vi "Main.vi"() -> ()   [LabVIEW 2013]
uses:
  <vilib>/myRIO/Instrument Drivers/Onboard IO/I2C/typedefs/I2C User Configuration.ctl
  <vilib>/myRIO/Instrument Drivers/Onboard IO/I2C/typedefs/I2C Transfer Rate.ctl
  <vilib>/Platform/TimedLoop/XDataNode/timing_clust.ctl
  <vilib>/Platform/TimedLoop/XDataNode/nitl_modes.ctl
  <vilib>/Platform/TimedLoop/XDataNode/wakeup.ctl
  <vilib>/myRIO/Common/Instrument Driver Framework/myRIO v1.0/DIO/vis/myRIO v1.1 Open DIO.vi
  <vilib>/myRIO/Common/Instrument Driver Framework/myRIO v1.0/I2C/vis/myRIO v1.1 Open I2C.vi
  <vilib>/myRIO/Common/Instrument Driver Framework/myRIO v1.0/UART/vis/myRIO v1.0 Close UART.vi
  <vilib>/myRIO/Common/Instrument Driver Framework/Utilities/vis/Validate Channels.vi
  <vilib>/myRIO/Common/Instrument Driver Framework/myRIO v1.0/DIO/vis/myRIO v1.0 Reserve DIO.vi
  <vilib>/myRIO/Common/Instrument Driver Framework/myRIO v1.0/I2C/vis/myRIO v1.0 Reserve I2C.vi
  <vilib>/myRIO/Common/Instrument Driver Framework/myRIO v1.0/Resource Manager/vis/myRIO v1.0 Reserve Channel List.vi
  <vilib>/myRIO/Common/Instrument Driver Framework/myRIO v1.0/DIO/vis/myRIO v1.0 Build MUX Configuration DIO.vi
  <vilib>/myRIO/Common/Instrument Driver Framework/myRIO v1.0/I2C/vis/myRIO v1.0 Build MUX Configuration I2C.vi
  <vilib>/myRIO/Common/Instrument Driver Framework/myRIO v1.0/Resource Manager/vis/myRIO v1.0 Reserve Channel.vi
  <vilib>/myRIO/Common/Instrument Driver Framework/myRIO v1.0/Resource Manager/vis/myRIO v1.0 Unreserve Channel.vi
  <vilib>/myRIO/Common/Instrument Driver Framework/myRIO v1.0/Resource Manager/vis/myRIO v1.0 Create Configuration List.vi
  <vilib>/myRIO/Common/Instrument Driver Framework/myRIO v1.0/Resource Manager/vis/myRIO v1.0 Build Mutex Name.vi
  <vilib>/myRIO/Common/Instrument Driver Framework/myRIO v1.0/myRIO v1.1 Open.vi
  <vilib>/Utility/VariantDataType/GetNumericInfo.vi
  <vilib>/Utility/error.llb/Error Cluster From Error Code.vi
  <vilib>/myRIO/Common/Instrument Driver Framework/Utilities/vis/IO Manager.vi
  <vilib>/myRIO/Common/Instrument Driver Framework/Utilities/vis/Configuration Manager.vi
  <vilib>/myRIO/Common/Instrument Driver Framework/myRIO v1.0/Resource Manager/vis/myRIO v1.0 Configure IO.vi
  <vilib>/myRIO/Common/Instrument Driver Framework/myRIO v1.0/myRIO v1.0 Close.vi
  <vilib>/myRIO/Common/Instrument Driver Framework/myRIO v1.0/I2C/vis/myRIO v1.0 Configure I2C.vi
  <vilib>/myRIO/Common/Instrument Driver Framework/myRIO v1.0/I2C/vis/myRIO v1.0 Write I2C.vi
  <vilib>/myRIO/Common/Instrument Driver Framework/myRIO v1.0/DIO/vis/myRIO v1.0 Read DIO.vi
  <vilib>/myRIO/Common/Instrument Driver Framework/myRIO v1.0/DIO/vis/myRIO v1.0 Write DIO.vi
  <vilib>/myRIO/Common/Instrument Driver Framework/myRIO v1.0/I2C/vis/myRIO v1.0 Read I2C.vi
  <vilib>/myRIO/Common/Instrument Driver Framework/Utilities/vis/FPGA Ref Manager.vi
  <vilib>/myRIO/Common/Instrument Driver Framework/myRIO v1.0/myRIO v1.0 Reset FPGA.vi
  <vilib>/platform/TimedLoop/XDataNode/XDataNode.xnode
  <vilib>/myRIO/Instrument Drivers/Utilities/Utilities.lvlib
  <vilib>/myRIO/Instrument Drivers/Onboard IO/I2C/I2C.lvlib
  <vilib>/myRIO/Instrument Drivers/Onboard IO/DIO/DIO.lvlib
  <vilib>/Platform/TimedLoop/XDataNode/XDNodeRunTimeDep.lvlib
panel:
  out "INT_SOURCE":bool[](array[boolean])
  out "Waveform Chart":cluster{i16, i16, i16}(graph)
  out "DATA":u8[](array[numeric]) format="%02x"
  out "Z":i16
  out "Y":i16
  out "X":i16
  in  "[ESC]":bool
  # "Accelerometer demo"
  # "DATAX0"
  # "DATAX1"
  # "DATAY0"
  # "DATAY1"
  # "DATAZ0"
  # "DATAZ1"
  # "D = data ready\n1T = single-tap\n2T = double-tap"
  # "A = activity\nI = inactivity\nF = free fall"
  # "W = watermark\nO = overrun"
  # "D   1T  2T   A    I     F    W   O"
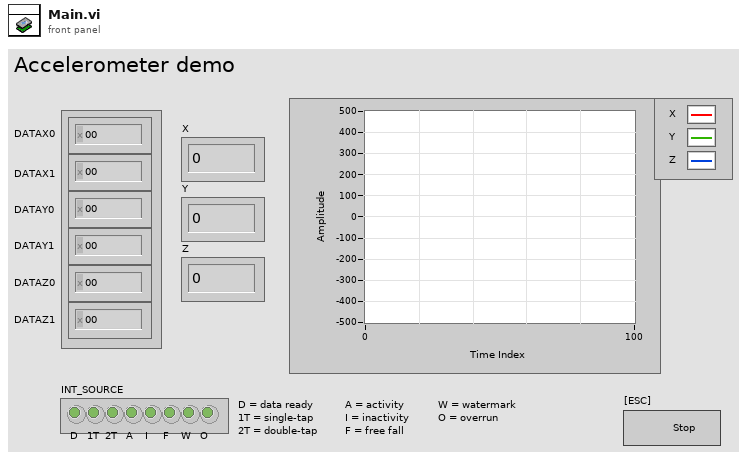
[diagram p1: front panel]
types:
  T1 = typedef "I2C.lvlib/I2C User Configuration.ctl" = cluster{"I2C Transfer Rate":T2}
  T2 = typedef "I2C.lvlib/I2C Transfer Rate.ctl" = enum16{"Standard Mode (100 kbps)", "Fast Mode (400 kbps)"}
  T3 = typedef "I2C.lvlib/I2C Reference.ctl" = cluster{"myRIO Reference":T4, "I2C Channels Enum":T8, "I2C Configuration":T9}
  T4 = typedef "myRIO Generic Hardware Reference.ctl" = cluster{"myRIO Model":T5, "myRIO Hardware Reference":T6}
  T5 = typedef "Hardware Version Enum.ctl" = enum16{"Unknown", "myRIO-1900", "myRIO-1950"}
  T6 = typedef "myRIO v1.0 Reference.ctl" = cluster{"Generic FPGA Reference":T7, "Allow multiple opens":bool}
  T7 = typedef "Generic FPGA Reference.ctl" = refnum<k20>
  T8 = typedef "I2C Channels Enum.ctl" = enum16{"Not Connected", "A/I2C", "B/I2C"}
  T9 = typedef "I2C.lvlib/I2C Configuration.ctl" = cluster{"I2C Transfer Rate":T2}
  T10 = typedef "DIO.lvlib/DIO Reference.ctl" = cluster{"myRIO Reference":T4, "DIO Channels List":T11}
  T11 = typedef "DIO Channels List.ctl" = T12[]
  T12 = typedef "DIO Channels Enum.ctl" = enum16{"Not Connected", "C/DIO0", "C/DIO1", "C/DIO2", "C/DIO3", "C/DIO4", "C/DIO5", "C/DIO6", "C/DIO7", "A/DIO0", "A/DIO1", "A/DIO2", "A/DIO3", "A/DIO4", "A/DIO5", "A/DIO6", "A/DIO7", "A/DIO8", "A/DIO9", "A/DIO10", "A/DIO11", "A/DIO12", "A/DIO13", "A/DIO14", "A/DIO15", "B/DIO0", "B/DIO1", "B/DIO2", "B/DIO3", "B/DIO4", "B/DIO5", "B/DIO6", "B/DIO7", "B/DIO8", "B/DIO9", "B/DIO10", "B/DIO11", "B/DIO12", "B/DIO13", "B/DIO14", "B/DIO15", "LED0", "LED1", "LED2", "LED3", "Button0"}
  T13 = typedef "XDNodeRunTimeDep.lvlib/timing_clust.ctl" = cluster{"Expected End [f-1]":u64, "Actual End [f-1]":u64, "Finished Late? [f-1]":bool, "Expected End [i-1]":u64, "Actual End [i-1]":u64, "Finished Late? [i-1]":bool, "Expected Start [i]":u64, "Actual Start [i]":u64, "Expected Start [f]":u64, "Actual Start [f]":u64, "Source Name":string, "Structure Name":string, "Period":i64, "Deadline":i64, "Offset":i64, "Start":i64, "Priority":i32, "Timeout":i32, "Mode":T14, "Wakeup Reason":T15, "Error":errorcluster, "Source Type":string, "Secondary Source Type":string, "Global End Time":u64, "Global Start Time":u64, "Frame Duration":u64, "Iteration Duration":u64, "Assigned CPU":i32, "I/O Scan Engine Mode":u32}
  T14 = typedef "XDNodeRunTimeDep.lvlib/nitl_modes.ctl" = enum32{"No Change", "Process missed periods, maintain original phase", "Discard missed periods, maintain original phase", "Process missed periods, ignore original phase", "Discard missed periods, ignore original phase"}
  T15 = typedef "XDNodeRunTimeDep.lvlib/wakeup.ctl" = enum32{"Normal", "Aborted", "Asynchronous wakeup", "Timing source error", "Timed loop error", "Timeout"}
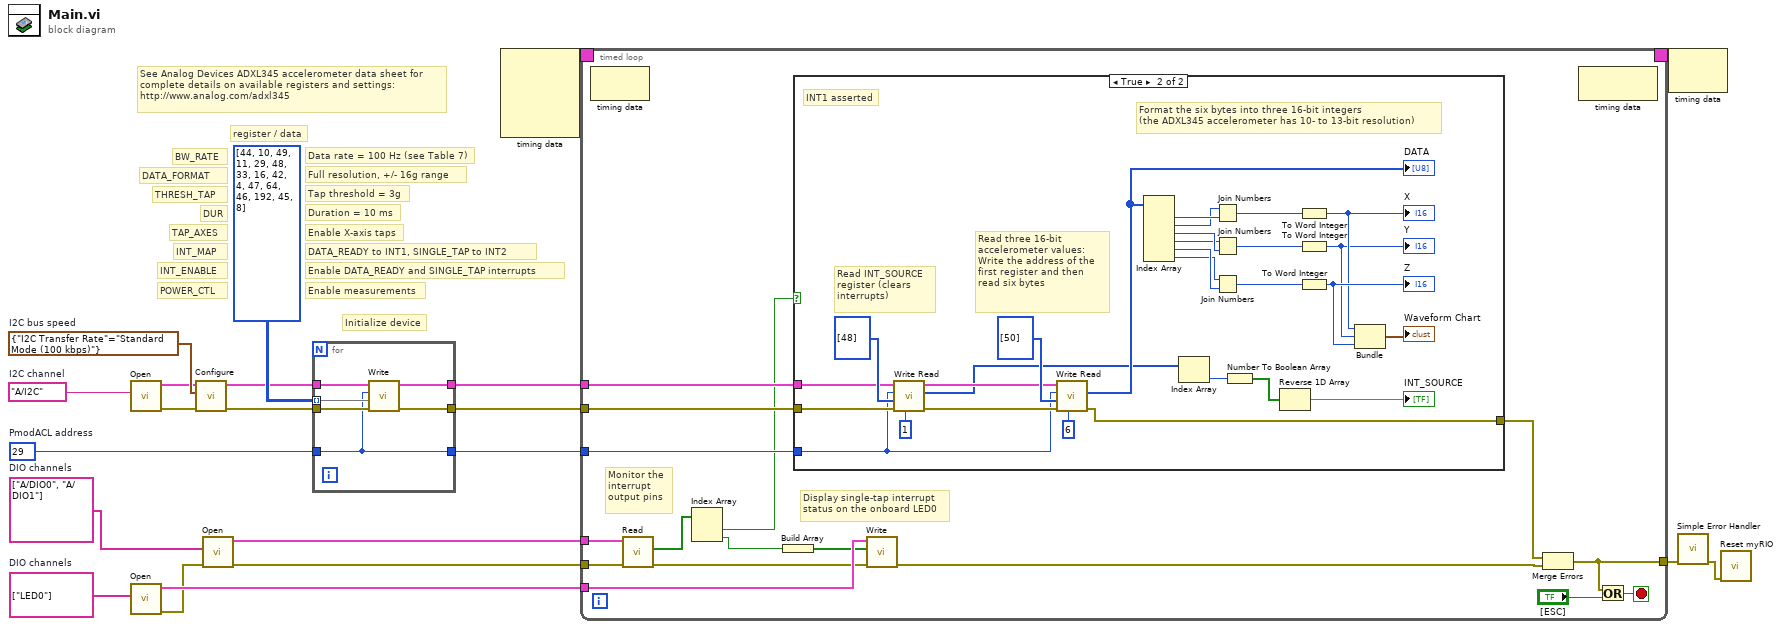
[diagram p0: block diagram]
diagram:
  w3 = tag[] ["LED0"]  # DIO channels
  w6 = tag[] ["A/DIO0", "A/DIO1"]  # DIO channels
  w18 = T1 {"I2C Transfer Rate"=enum."Standard Mode (100 kbps)"}  # I2C bus speed
  w19 = tag "A/I2C"  # I2C channel
  w9 = u8 29  # PmodACL address
  # "Data rate = 100 Hz (see Table 7)"
  # "BW_RATE"
  # "DATA_READY to INT1, SINGLE_TAP to INT2"
  # "INT_MAP"
  # "Enable X-axis taps"
  # "TAP_AXES"
  # "Initialize device"
  # "Enable measurements"
  # "Enable DATA_READY and SINGLE_TAP interrupts"
  # "Duration = 10 ms"
  # "Tap threshold = 3g"
  # "See Analog Devices ADXL345 accelerometer data sheet for\ncomplete details on available registers and settings:\nhttp://www.analog.com/adxl345"
  # "POWER_CTL"
  # "INT_ENABLE"
  # "DUR"
  # "THRESH_TAP"
  # "Full resolution, +/- 16g range"
  # "DATA_FORMAT"
  # "register / data"
  n1 = call <vilib>:"Open.vi"("Channel Name"=w19) -> ("error out"=w16:errorcluster, "I2C Ref Out"=w17:T3)  [unwired: 9 in]
  n2 = call <vilib>:"Open.vi"("Channel Names"=w3) -> ("error out"=w1:errorcluster, "DIO Ref Out"=w2:T10)  [unwired: 9 in]
  n3 = call <vilib>:"Configure.vi"("error in (no error)"=w16, "I2C User Configuration"=w18, "I2C Ref In"=w17) -> ("error out"=w10:errorcluster, "I2C Ref Out"=w11:T3)  [unwired: 7 in]
  n4 = call <vilib>:"Open.vi"("error in (no error)"=w1, "Channel Names"=w6) -> ("error out"=w8:errorcluster, "DIO Ref Out"=w7:T10)  [unwired: 8 in]
  n5 = for {
    tunnel: [w27] -> w15
    tunnel: [w26] -> w14
    tunnel: [w22] -> w13
    tunnel: u8[][] [[44, 10], [49, 11], [29, 48], [33, 16], [42, 4], [47, 64], [46, 192], [45, 8]] ("Bytes to Write") -> [w25] mode=indexing
    tunnel: w11 -> [w24]
    tunnel: w10 -> [w23]
    tunnel: w9 -> [w22]
    n6 = call <vilib>:"Write.vi"("error in (no error)"=w23, "Bytes to Write"=w25, "Slave Address (7-bit)"=w22, "I2C Ref In"=w24) -> ("error out"=w27:errorcluster, "I2C Ref Out"=w26:T3)  [unwired: 6 in]
  }
  n7 = node-c288() -> (w5:T13)  [unwired: 4 in]
  n8 = timed-loop {
    tunnel: [w28] -> w20
    tunnel: w13 -> [w39]
    tunnel: w15 -> [w41]
    tunnel: w14 -> [w40]
    tunnel: w8 -> [w38]
    tunnel: w7 -> [w37]
    timing: w5 -> [_]
    timing-out: [_] -> w4
    tunnel: w2 -> [w33]
    stop <- w43 stop-if-true
    # "Display single-tap interrupt\nstatus on the onboard LED0"
    # "Monitor the\ninterrupt\noutput pins"
    n9 = node-c288() -> ()  [unwired: 1 in, 1 out]
    n10 = call <vilib>:"Read.vi"("error in (no error)"=w38, "DIO Ref In"=w37) -> ("error out"=w32:errorcluster, "Values"=w34:bool[])  [unwired: 7 in, 1 out]
    n11 = Index Array "Index Array"(array=w34) -> (element #1=w35:bool, element #2=w30:bool)  [unwired: 2 in]
    n12 = Build Array "Build Array"(w30) -> (w31:bool[])
    n13 = case shown="True" w35 {
      tunnel: w41 -> [w46 w65]
      tunnel: w40 -> [_ w64]
      tunnel: w39 -> [_ w53]
      tunnel: [w46 w49] -> w36
      frame False {
        # "INT1 deasserted"
      }
      frame True {
        # "INT1 asserted"
        # "Read INT_SOURCE\nregister (clears\ninterrupts)"
        # "Read three 16-bit accelerometer values:\nWrite the address of the first register and then read six bytes"
        # "Format the six bytes into three 16-bit integers\n(the ADXL345 accelerometer has 10- to 13-bit resolution)"
        n14 = call <vilib>:"Write Read.vi"("Byte Count"=u32 1, "error in (no error)"=w65, "Bytes to Write"=u8[] [48], "Slave Address (7-bit)"=w53, "I2C Ref In"=w64) -> ("error out"=w54:errorcluster, "Bytes Read"=w47:u8[], "I2C Ref Out"=w55:T3)  [unwired: 3 in]
        n15 = call <vilib>:"Write Read.vi"("Byte Count"=u32 6, "error in (no error)"=w54, "Bytes to Write"=u8[] [50], "Slave Address (7-bit)"=w53, "I2C Ref In"=w55) -> ("error out"=w49:errorcluster, "Bytes Read"=w48:u8[])  [unwired: 3 in, 1 out]
        "DATA" <- w48
        n16 = Index Array "Index Array"(array=w48) -> (element #1=w63:u8, element #2=w62:u8, element #3=w61:u8, element #4=w60:u8, element #5=w59:u8, element #6=w58:u8)  [unwired: 6 in]
        n17 = Index Array "Index Array"(array=w47) -> (element=w52:u8)  [unwired: 1 in]
        n18 = Join Numbers(hi=w62, lo=w63) -> ((hi.lo)=w74:u16)
        n19 = Join Numbers(hi=w60, lo=w61) -> ((hi.lo)=w73:u16)
        n20 = Join Numbers(hi=w58, lo=w59) -> ((hi.lo)=w72:u16)
        n21 = Number To Boolean Array(number=w52) -> (Boolean array=w51:bool[])
        n22 = Reverse 1D Array(array=w51) -> (reversed array=→"INT_SOURCE":bool[])
        n23 = To Word Integer(number=w74) -> (16bit integer=w69:i16)
        "X" <- w69
        n24 = To Word Integer(number=w73) -> (16bit integer=w68:i16)
        "Y" <- w68
        n25 = To Word Integer(number=w72) -> (16bit integer=w71:i16)
        "Z" <- w71
        n26 = Bundle "Bundle"(w69, w68, w71) -> (→"Waveform Chart":cluster{i16, i16, i16})  [unwired: 1 in]
      }
    }
    n27 = call <vilib>:"Write.vi"("error in (no error)"=w32, "Values"=w31, "DIO Ref In"=w33) -> ("error out"=w29:errorcluster)  [unwired: 6 in, 1 out]
    n28 = Merge Errors "Merge Errors"(w36, w29) -> (w28:errorcluster)
    n29 = node-c288() -> ()  [unwired: 1 in, 1 out]
    n30 = Or(x=w28, y="[ESC]") -> (x .or. y?=w43:bool)
  }
  n31 = node-c288(w4) -> ()  [unwired: 1 out]
  n32 = call <vilib>:"Simple Error Handler.vi"("error in (no error)"=w20) -> ("error out"=w21:errorcluster)  [unwired: 4 in, 4 out]
  n33 = call <vilib>:"Reset myRIO.vi"("error in (no error)"=w21) -> ()  [unwired: 10 in, 1 out]
